vi "Compression_Simulation_Get PAEs.vi"(6 "Adjusting Factor":dbl, 11 "POUTs in":dbl[](array[numeric])) -> (3 "PAEs out":dbl[](array[numeric]))   [LabVIEW 2023]
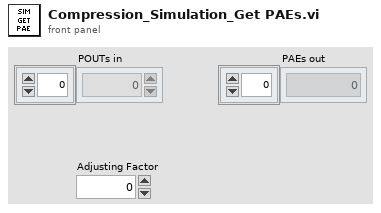
[diagram p1: front panel]
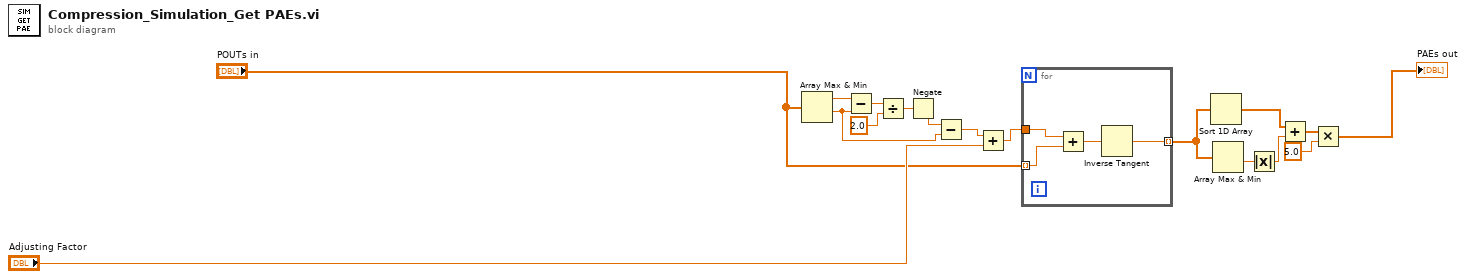
[diagram p0: block diagram]
diagram:
  n1 = Array Max & Min(array="POUTs in") -> (max value=w12:dbl, min value=w13:dbl)  [unwired: 2 out]
  n2 = Subtract(x=w12, y=w13) -> (x-y=w10:dbl)
  n3 = Divide(x=w10, y=2.0) -> (x/y=w9:dbl)
  n4 = Negate(x=w9) -> (-x=w14:dbl)
  n5 = Subtract(x=w14, y=w13) -> (x-y=w15:dbl)
  n6 = Add(x=w15, y="Adjusting Factor") -> (x+y=w16:dbl)
  n7 = for {
    tunnel: "POUTs in" -> [w19] mode=indexing
    tunnel: [w21] -> w5 mode=indexing
    tunnel: w16 -> [w20]
    n8 = Add(x=w20, y=w19) -> (x+y=w18:dbl)
    n9 = Inverse Tangent(1:w18) -> (0:w21:dbl)
  }
  n10 = Sort 1D Array(array=w5) -> (sorted array=w6:dbl[])
  n11 = Array Max & Min(array=w5) -> (min value=w2:dbl)  [unwired: 3 out]
  n12 = Absolute Value(x=w2) -> (abs(x)=w3:dbl)
  n13 = Add(x=w6, y=w3) -> (x+y=w1:dbl[])
  n14 = Multiply(x=w1, y=5.0) -> (x*y=→"PAEs out":dbl[])
